vi "KepcoDCPwr Query Dwell Count.vi"(0 "VISA Session":refnum<visa-resource-name>, 5 "Model In":string, 7 "channel name (\"\")":string="\"\"", 11 "error in (no error)":errorcluster {"code" format="%.0x"}) -> (4 "VISA Session Out":refnum<visa-resource-name>, 6 "Model Out":string, 8 "channel name out (\"\")":string="\"\"" caption="channel name Out (\"\")", 10 "voltage level":i32 caption="Dwell", 15 "error out":errorcluster {"code" format="%.0x"})   [LabVIEW 2013]
doc: "This VI returns the number of dwell points in use in a list."
uses:
  <vilib>/regexp/Match Regular Expression.xnode
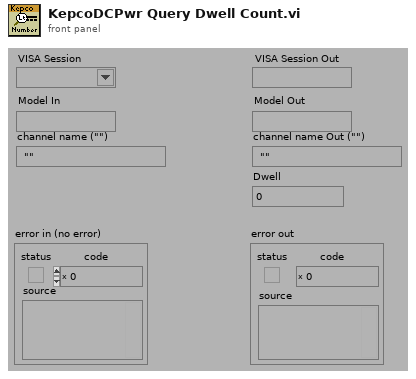
[diagram p1: front panel]
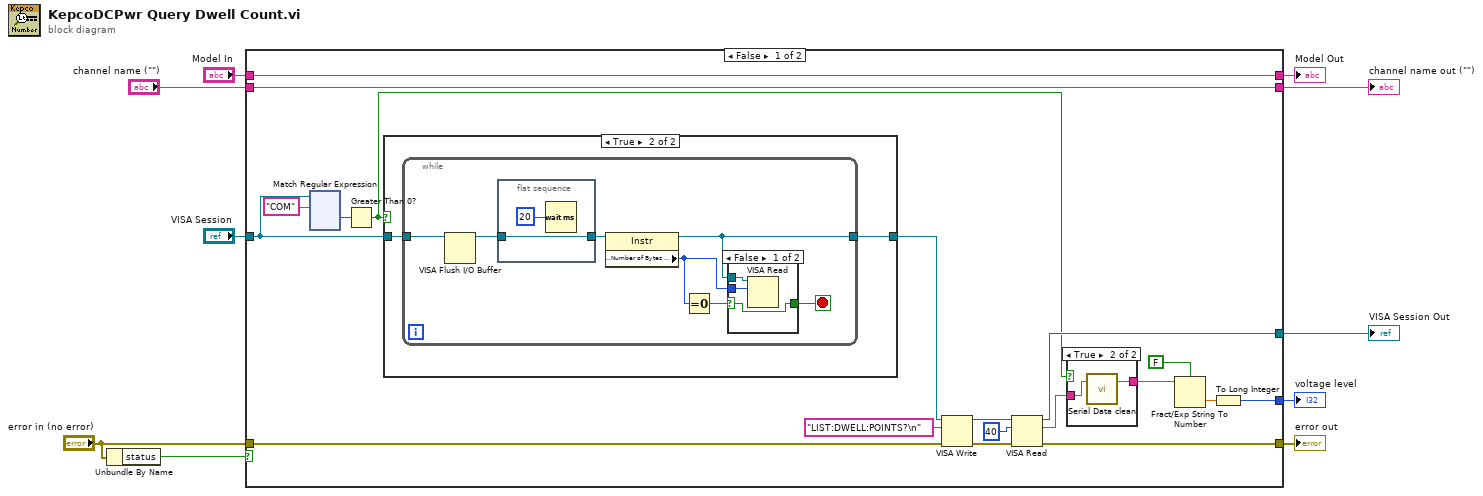
[diagram p0: block diagram]
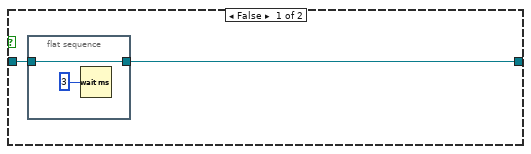
[diagram p3: hidden frame]
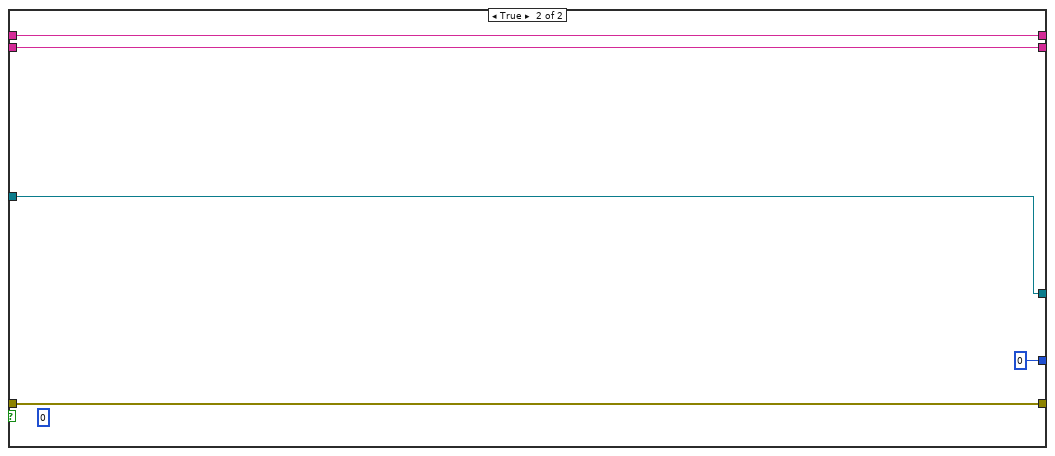
[diagram p5: hidden frame]
diagram:
  n1 = Unbundle By Name("error in (no error)") -> ("status"=w9:bool)
  n2 = case shown="False" w9 {
    tunnel: [w25 w167] -> w10
    tunnel: "error in (no error)" -> [w28 w167]
    tunnel: [w26 w166] -> w4
    tunnel: "VISA Session" -> [w20 w166]
    tunnel: [w27 w165] -> w3
    tunnel: "Model In" -> [w27 w165]
    tunnel: [w29 w164] -> w2
    tunnel: "channel name (\"\")" -> [w29 w164]
    tunnel: [w11 0] -> w1
    frame False {
      n3 = xnode "Match Regular Expression"("input string"=w20, "regular expression"="COM") -> ("offset past match"=w23:i32)  [unwired: 2 in, 6 out]
      n4 = Greater Than 0?(x=w23) -> (x > 0?=w22:bool)
      n5 = case shown="True" w22 {
        tunnel: [w34 w38] -> w21
        tunnel: w20 -> [w33 w37]
        frame False {
          n6 = flat-sequence {
            tunnel: w33 -> [w36]
            tunnel: [w36] -> w34
            frame #0 {
              n7 = Wait (ms)(milliseconds to wait=u32 3 ("byte count (0)")) -> ()  [unwired: 1 out]
            }
          }
        }
        frame True {
          n8 = while {
            tunnel: w37 -> [w41]
            tunnel: [w43] -> w38
            stop <- w44 stop-if-true
            n9 = VISA Flush I/O Buffer(VISA resource name=w41) -> (VISA resource name out=w40:refnum<visa-resource-name>)  [unwired: 2 in, 1 out]
            n10 = flat-sequence {
              tunnel: w40 -> [w46]
              tunnel: [w46] -> w39
              frame #0 {
                n11 = Wait (ms)(milliseconds to wait=u32 20) -> ()  [unwired: 1 out]
              }
            }
            n12 = property class="Instr"(reference=w39) -> (reference out=w43:refnum<visa-resource-name>, "Serial Settings:Number of Bytes at Serial Port"=w42:u32)  [unwired: 1 in, 1 out]
            n13 = Equal To 0?(x=w42) -> (x = 0?=w45:bool)
            n14 = case shown="False" w45 {
              selector: w45 -> [w50 w51]
              tunnel: [w50 w51] -> w44
              tunnel: w43 -> [w49 _]
              tunnel: w42 -> [w48 _]
              frame False {
                n15 = VISA Read(VISA resource name=w49, byte count=w48) -> ()  [unwired: 1 in, 4 out]
              }
              frame True {
              }
            }
          }
        }
      }
      n16 = VISA Write(VISA resource name=w21, write buffer="LIST:DWELL:POINTS?\n", error in (no error)=w28) -> (VISA resource name out=w17:refnum<visa-resource-name>, error out=w16:errorcluster)  [unwired: 1 out]
      n17 = VISA Read(VISA resource name=w17, byte count=u32 40 ("byte count (0)"), error in (no error)=w16) -> (VISA resource name out=w26:refnum<visa-resource-name>, read buffer=w15:string, error out=w25:errorcluster)  [unwired: 1 out]
      n18 = case shown="True" w22 {
        tunnel: w15 -> [w30 w31]
        tunnel: [w30 w32] -> w14
        frame False {
        }
        frame True {
          n19 = call "Serial Data clean.vi"("string"=w31) -> ("Stripped of Xon Xoff"=w32:string)  [unwired: 2 in]
        }
      }
      n20 = Fract/Exp String To Number(use system decimal point (T)=FALSE, string=w14) -> (number=w12:dbl)  [unwired: 2 in, 1 out]
      n21 = To Long Integer(number=w12) -> (32bit integer=w11:i32)
    }
    frame True {
      (unwired) 0
    }
  }
  "error out" <- w10
  "channel name out (\"\")" <- w2
  "Model Out" <- w3
  "VISA Session Out" <- w4
  "voltage level" <- w1
